vi "1.3 Producer Consumer Test but with channel wires.vi"() -> ()   [LabVIEW 2018]
uses:
  <vilib>/DAQmx/read.llb/DAQmx Read (Analog DBL 1Chan 1Samp).vi
  <extravilib>/ChannelInstances/Stream-dbl/Read With Abort.vi
  <extravilib>/ChannelInstances/Stream-dbl/Write With Abort.vi
  <extravilib>/ChannelInstances/Stream-dbl/EndpointRead.vi
  <extravilib>/ChannelInstances/Stream-dbl/Endpoint.vi
  <vilib>/DAQmx/create/channels.llb/DAQmx Create Channel (AI-Voltage-Basic).vi
  <vilib>/DAQmx/configure/timing.llb/DAQmx Timing (Sample Clock).vi
  <extravilib>/ChannelInstances/Stream-dbl/Instantiate.vi
  <extravilib>/ChannelInstances/Stream-dbl/)Channel.vi
  <resource>/ChannelSupport/_ChannelSupport/WaitIfNeeded.vi
  <vilib>/DAQmx/miscellaneous.llb/DAQmx Fill In Error Info.vi
  <extravilib>/ChannelInstances/Stream-dbl.lvlib
panel:
  in  "Average of ?":dbl
  out "Data saving loop 2":dbl(graph)
  in  "Boolean":bool
  in  "stop 2":bool
  out "Data saving loop":dbl(graph)
  out "Producer Data":dbl(graph)
  in  "stop":bool
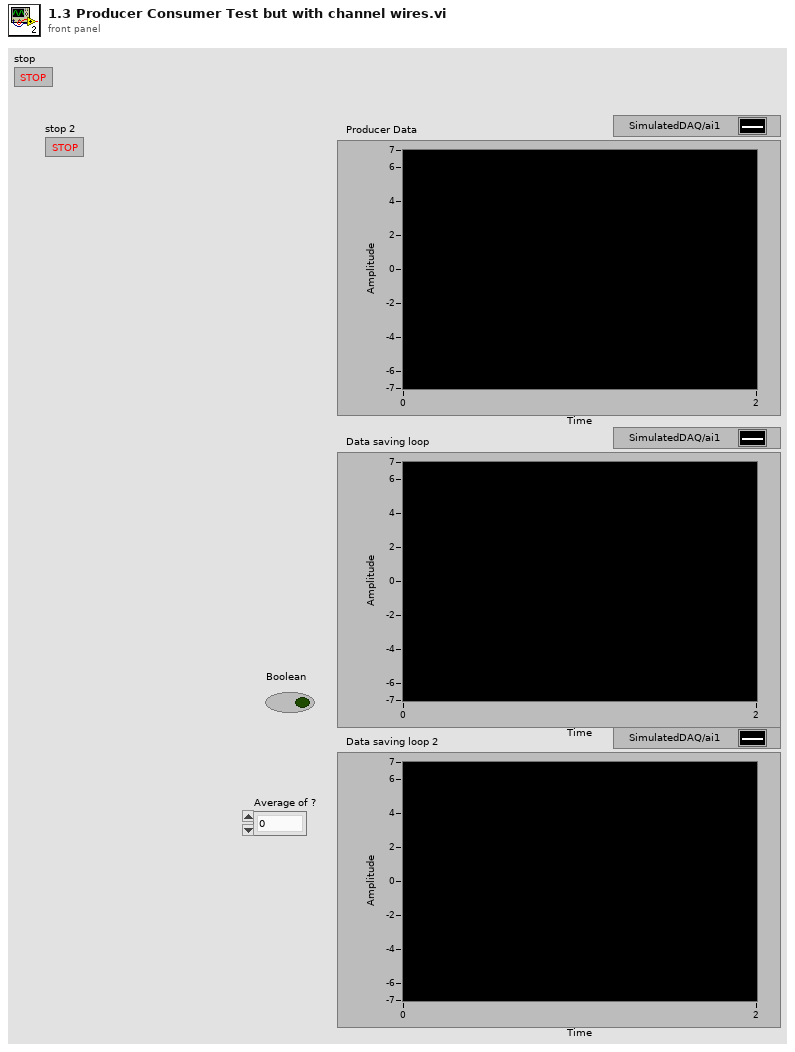
[diagram p1: front panel]
types:
  T1 = typedef "Stream-dbl.lvlib/)Channel.ctl" = refnum<queue>
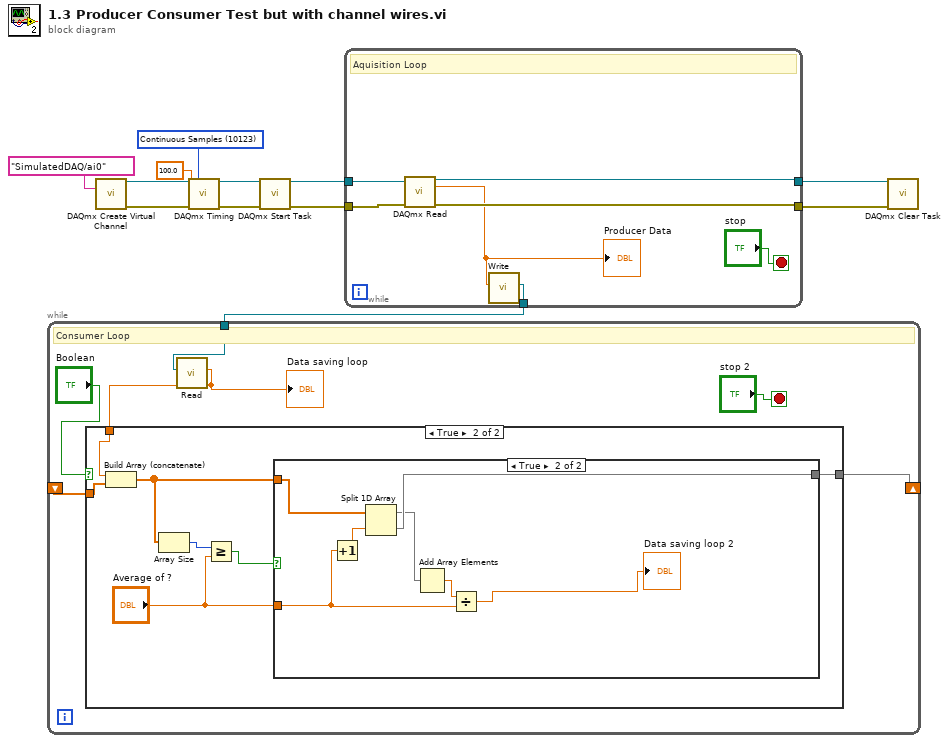
[diagram p0: block diagram]
diagram:
  w8 = 10123 items=["Finite Samples"=10178, "Continuous Samples"=10123, "Hardware Timed Single Point"=12522] ("sample mode")
  n1 = call-poly <vilib>:"DAQmx Create Virtual Channel.vi"("physical channels"=tag "SimulatedDAQ/ai0") -> ("task out"=w9:refnum<k21>, "error out"=w10:errorcluster)  [unwired: 13 in]
  n2 = call-poly <vilib>:"DAQmx Timing.vi"("task/channels in"=w9, "sample mode"=w8, "rate"=100.0, "error in"=w10) -> ("task out"=w11:refnum<k21>, "error out"=w12:errorcluster)  [unwired: 10 in]
  n3 = call <vilib>:"DAQmx Start Task.vi"("task/channels in"=w11, "error in"=w12) -> ("task out"=w2:refnum<k21>, "error out"=w3:errorcluster)  [unwired: 12 in]
  n4 = while {
    tunnel: w2 -> [w15]
    tunnel: w3 -> [w18]
    tunnel: [w17] -> w6
    tunnel: [w16] -> w5
    tunnel: [w13] -> w1
    stop <- "stop" stop-if-true
    # "Aquisition Loop"
    n5 = call-poly <vilib>:"DAQmx Read.vi"("task/channels in"=w15, "error in"=w18) -> ("task out"=w17:refnum<k21>, "data"=w14:dbl, "error out"=w16:errorcluster)  [unwired: 11 in]
    "Producer Data" <- w14
    n6 = call <extravilib>:"Write.vi"("element"=w14) -> ("channel"=w13:T1)  [unwired: 8 in, 2 out]
  }
  n7 = while {
    shift-right: [w20] -> _
    shift-left: _ -> [w25]
    tunnel: w1 -> [w24]
    stop <- "stop 2" stop-if-true
    # "Consumer Loop"
    n8 = call <extravilib>:"Read.vi"("channel"=w24) -> ("element"=w23:dbl)  [unwired: 6 in, 4 out]
    "Data saving loop" <- w23
    n9 = case shown="True" "Boolean" {
      tunnel: w25 -> [w26 w31]
      tunnel: w23 -> [_ w33]
      tunnel: [w26 w32] -> w20
      frame False {
      }
      frame True {
        n10 = Build Array (concatenate)(w33, w31) -> (w30:dbl[])
        n11 = Array Size(array=w30) -> (size(s)=w29:i32)
        n12 = Greater Or Equal?(x=w29, y="Average of ?") -> (x >= y?=w28:bool)
        n13 = case shown="True" w28 {
          tunnel: [w34 w40] -> w32
          tunnel: w30 -> [w34 w41]
          tunnel: "Average of ?" -> [_ w35]
          frame False {
          }
          frame True {
            n14 = Increment(x=w35) -> (x+1=w36:dbl)
            n15 = Split 1D Array(array=w41, index=w36) -> (first subarray=w39:dbl[], second subarray=w40:dbl[])
            n16 = Add Array Elements(numeric array=w39) -> (sum=w38:dbl)
            n17 = Divide(x=w38, y=w35) -> (x/y=→"Data saving loop 2":dbl)
          }
        }
      }
    }
  }
  n18 = call <vilib>:"DAQmx Clear Task.vi"("task in"=w6, "error in"=w5) -> ()  [unwired: 13 in, 1 out]
